vi "Register An Assert VI.vi"(8 "error in (no error)":errorcluster, 11 "first call?":bool) -> (0 "error out":errorcluster)   [LabVIEW 2013, in "Caraya.lvlib" / "Assert.lvclass"]
doc: "Call this VI from the block diagram of a VI to register that VI as an assert VI. Typically, the Boolean input is connected to a <b>First Call?</b> node. Registering the VI makes Caraya consider the VI to be part of the assert framework and not part of the user's test code for the purposes of reporting call chains. \n\nThis VI executes even if there is an error passed to the <b>error in</b> terminal."
uses:
  Assert.lvclass
  Registry For Assert VIs.vi
  <vilib>/regexp/Match Regular Expression.xnode
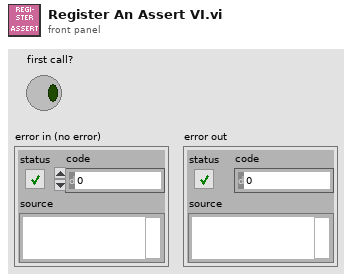
[diagram p1: front panel]
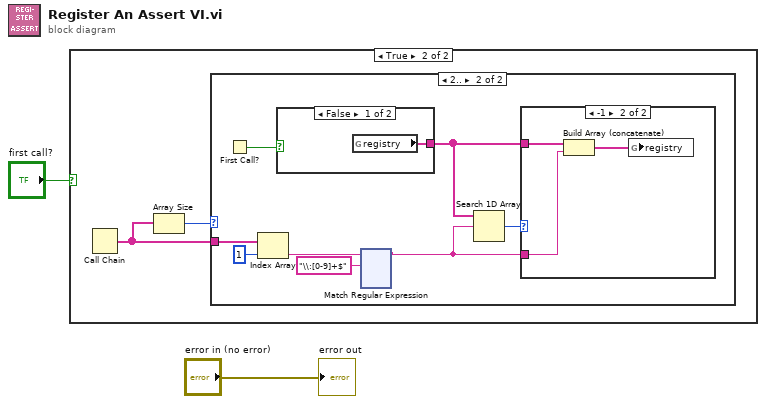
[diagram p0: block diagram]
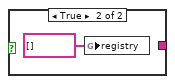
[diagram p4: hidden frame]
diagram:
  n1 = case shown="True" "first call?" {
    frame False {
    }
    frame True {
      n2 = Call Chain() -> (call chain=w3:string[])
      n3 = Array Size(array=w3) -> (size(s)=w4:i32)
      n4 = case shown="2.." w4 {
        tunnel: w3 -> [_ w12]
        frame Default {
        }
        frame 2.. {
          n5 = First Call?() -> (First Call?: T/F=w9:bool)
          n6 = Index Array(array=w12, index=1) -> (element=w7:string)
          n7 = case shown="False" w9 {
            tunnel: [w127 _] -> w8
            frame False {
              n8 = global read "Registry For Assert VIs.vi" "registry"() -> (w127:string[])
            }
            frame True {
              n9 = global write "Registry For Assert VIs.vi" "registry"(string[] [] ("registry")) -> ()
            }
          }
          n10 = xnode "Match Regular Expression"("input string"=w7, "regular expression"="\\:[0-9]+$") -> ("before match"=w5:string)  [unwired: 4 in, 4 out]
          n11 = Search 1D Array(1D array=w8, element=w5) -> (index of element=w10:i32)  [unwired: 1 in]
          n12 = case shown="-1" w10 {
            tunnel: w8 -> [_ w131]
            tunnel: w5 -> [_ w130]
            frame Default {
            }
            frame -1 {
              n13 = Build Array (concatenate)(w131, w130) -> (w129:string[])
              n14 = global write "Registry For Assert VIs.vi" "registry"(w129) -> ()
            }
          }
        }
      }
    }
  }
  "error out" <- "error in (no error)"
